vi "Get URI.vi"(11 "IRegister in":refnum<class "IRegister.lvclass">) -> (2 "URI":string, 3 "IRegister out":refnum<class "IRegister.lvclass">)   [LabVIEW 2020, in "wamplv.lvlib" / "IRegister.lvclass"]
uses:
  IRegister.lvclass
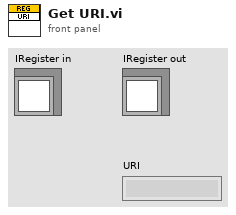
[diagram p1: front panel]
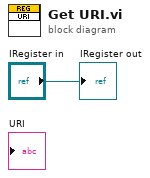
[diagram p0: block diagram]
diagram:
  "IRegister out" <- "IRegister in"
